vi "A_times_x_fxp.vi"(9 "Az_mat in":fxp<+/-,32,5>[][](array[numeric]), 10 "x_k":fxp<+/-,32,5>[](array[numeric])=[0.0, 0.0, 0.0, 0.0, 0.0, 0.0, 0.0, 0.0, 0.0, 0.0, 0.0, 0.0, 0.0, 0.0, 0.0, 0.0, 0.0, 0.0, 0.0, 0.0, 0.0, 0.0, 0.0, 0.0, 0.0, 0.0, 0.0, 0.0, 0.0, 0.0, 0.0, 0.0, 0.0, 0.0, 0.0, 0.0, 0.0, 0.0, 0.0, 0.0, 0.0, 0.0, 0.0, 0.0, 0.0, 0.0, 0.0, 0.0, 0.0, 0.0], 11 "NS":u8) -> (2 "A*x":fxp<+/-,64,12>[](array[numeric]), 3 "Az_vec out":fxp<+/-,32,5>[](array[numeric]))   [LabVIEW 2017, in "FXP_observer_TestCase.lvclass"]
uses:
  FXP_observer_TestCase.lvclass
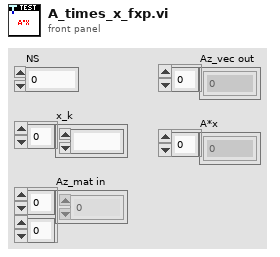
[diagram p1: front panel]
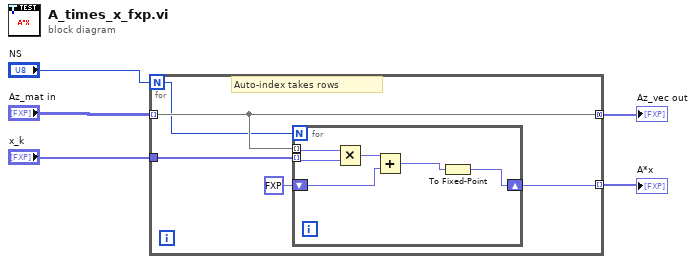
[diagram p0: block diagram]
diagram:
  n1 = for {
    N: "NS" -> [w6]
    tunnel: "Az_mat in" -> [w10] mode=indexing
    tunnel: [w10] -> w3 mode=concatenating
    tunnel: "x_k" -> [w9]
    tunnel: [w7] -> w4 mode=indexing
    # "Auto-index takes rows"
    n2 = for {
      N: w6 -> [_]
      tunnel: w10 -> [w16] mode=indexing
      tunnel: w9 -> [w15] mode=indexing
      shift-right: [w11] -> w7
      shift-left: fxp<+,1,1> 0.0 -> [w13]
      n3 = Multiply(x=w16, y=w15) -> (x*y=w14:fxp<+/-,64,10>)
      n4 = Add(x=w14, y=w13) -> (x+y=w12:fxp<+/-,64,13>)
      n5 = To Fixed-Point(number=w12) -> (fixed-point=w11:fxp<+/-,64,12>)  [unwired: 1 in]
    }
  }
  "A*x" <- w4
  "Az_vec out" <- w3
